vi "write project ref.vi"(10 "project ref":refnum<vi>, 11 "Builders in":refnum<class "Builder.lvclass">) -> (3 "Builders out":refnum<class "Builder.lvclass">)   [LabVIEW 2024, in "Builder.lvclass"]
uses:
  Builder.lvclass
  Builder.lvclass/Builder.ctl
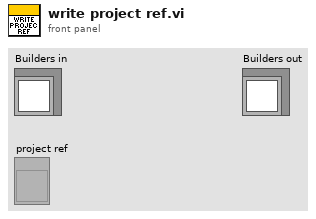
[diagram p1: front panel]
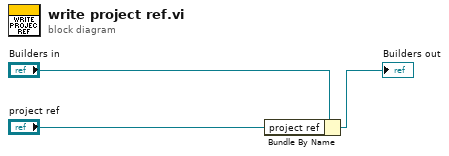
[diagram p0: block diagram]
diagram:
  n1 = Bundle By Name(cluster="Builders in", "project ref"="project ref") -> (→"Builders out":refnum<class "Builder.lvclass">)
